vi "fix.vi"(8 "error in (no error)":errorcluster, 10 "result":refnum<class "VideoFile.lvclass">, 11 "AudioMixer in":refnum<class "AudioMixer.lvclass">) -> (0 "error out":errorcluster, 2 "result out":refnum<class "VideoFile.lvclass">, 3 "AudioMixer out":refnum<class "AudioMixer.lvclass">)   [LabVIEW 2017, in "AudioMixer.lvclass"]
uses:
  AudioMixer.lvclass
  VideoFile Class/VideoFile.lvclass
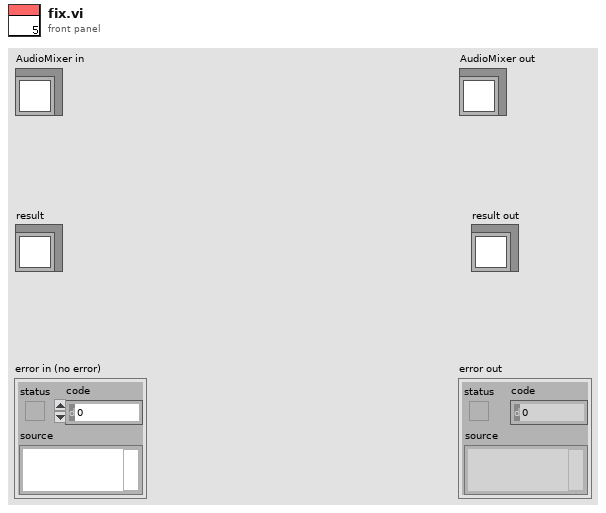
[diagram p1: front panel]
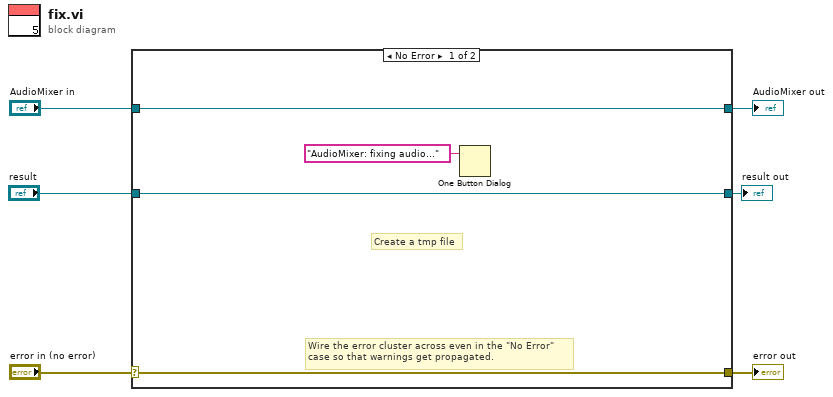
[diagram p0: block diagram]
diagram:
  n1 = case shown="No Error" "error in (no error)" {
    selector: "error in (no error)" -> [w9 w13]
    tunnel: [w9 w13] -> w5
    tunnel: [w10 w12] -> w3
    tunnel: "AudioMixer in" -> [w10 w12]
    tunnel: "result" -> [w7 w11]
    tunnel: [w7 w11] -> w1
    frame No Error {
      # "Create a tmp file"
      # "Wire the error cluster across even in the \"No Error\"\ncase so that warnings get propagated."
      n2 = One Button Dialog(message="AudioMixer: fixing audio...") -> ()  [unwired: 1 in, 1 out]
    }
    frame Error {
    }
  }
  "error out" <- w5
  "AudioMixer out" <- w3
  "result out" <- w1
